vi "Email Worker (Tester).vi"(10 "Message Cluster":T1, 11 "Send Email?":bool) -> ()   [LabVIEW 2019]
doc: "Assembles the components of the message cluster into a more human-friendly email body message. Passes this, a constructed subject line, and the distribution list the Send Email subvi"
uses:
  Globals and Definitions/Initialization Globals.vi
  a5bfeb0e-6229-4f50-a4ef-3b1ccf936079.vi
  Globals and Definitions/System Message.ctl
panel:
  out "Receipients":string[](array[string])
  out "Message Subject Line":string
  out "Message Body":string
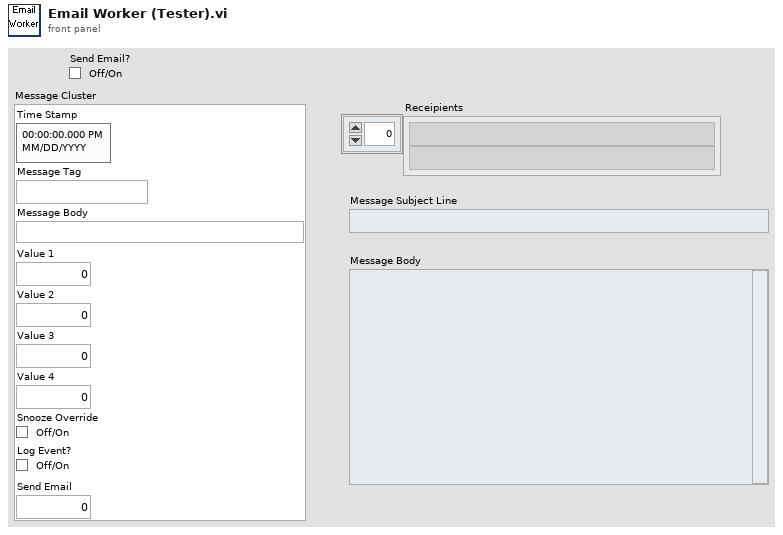
[diagram p1: front panel]
types:
  T1 = typedef "System Message.ctl" = cluster{"Time Stamp":timestamp, "Message Tag":string, "Message Body":string, "Value 1":i32, "Value 2":i32, "Value 3":dbl, "Value 4":dbl, "Snooze Override":bool, "Log Event?":bool, "Send Email":i32}
  T2 = typedef "All Tab Controls RDv1.0.ctl" = cluster{"Watch Circle":T3, "FTP and AWS":T4, "Email Settings":T5, "Summary File":T6, "File Settings":T7, "Watchdog":T9, "PowGrp0":T10, "Scaling Factors Grp0":dbl[], "PowGrp0 Sampling":cluster{"PowGrp0 sample rate [Hz]":dbl, "PowGrp0 samples per channel":i32}, "Stbd 3 Phase Voltage Scaling":dbl[], "Stbd 3 Phase Current Scaling":dbl[]}
  T3 = typedef "Watch Circle.ctl" = cluster{"Set Point Lat (dd)":dbl, "Set Point Lon (dd)":dbl, "Yellow Alert Radius (m)":dbl, "Red Alert Radius (m)":dbl, "AWOL Radius (m)":dbl, "Yellow Alert Snooze (min)":dbl, "Red Alert Snooze (min)":dbl, "AWOL Radius Snooze (min)":dbl}
  T4 = typedef "AWS and FTP.ctl" = cluster{"AWS Access Key":string, "AWS Secret Key":string, "AWS Bucket":string, "Enable AWS Upload (Summary)":bool, "Enable FTP Upload":bool, "FTP Host":string, "FTP User":string, "FTP Password":string, "Destination write path (pos)":string, "Local file path (pos)":string, "Summary  Upload Interval pos (min)":i32, "Delete Local File After Upload":bool, "Destination write path (pow)":string, "Local file path (pow)":string, "Summary Upload Interval pow (min)":i32, "Enable AWS Upload (TDMS)":bool}
  T5 = typedef "Email Settings.ctl" = cluster{"Enable Alerts":bool, "Distribution List (comma separated) 1":string, "Distribution List (comma separated) 2":string, "Sender Email":string, "SMTP":string, "Username":string, "Password":string}
  T6 = typedef "Summary File.ctl" = cluster{"Enable CSV":bool, "CSV Averaging Time (Sec)":i32, "CSV Loop Delay (ms)":i32}
  T7 = typedef "File Settings.ctl" = cluster{"Config File Path":string, "Data Folder Path":string, "Raw Mode":string, "Raw Interval (min)":i32, "Raw Sampling Time (min)":i32, "TDMS File Write Interval":T8, "Default Filename":path, "Enable TDMS Save (3ph only)":bool}
  T8 = typedef "Enum_FileNewInterval.ctl" = enum16{"10 Min", "Hourly", "Daily", "Weekly", "Monthly"}
  T9 = typedef "Watchdog.ctl" = cluster{"Watchdog Period (ms)":u32, "Reset System on WD timeout":bool, "Enable RT Watchdog":bool}
  T10 = typedef "TDMS Constants.ctl" = cluster{"Channel Names":string[], "Channel Units":string[], "TDMS File Suffix":string, "Channel Datatype":string[]}
  T11 = typedef "MODAQ _FPGA VI Reference.ctl" = refnum<k20>
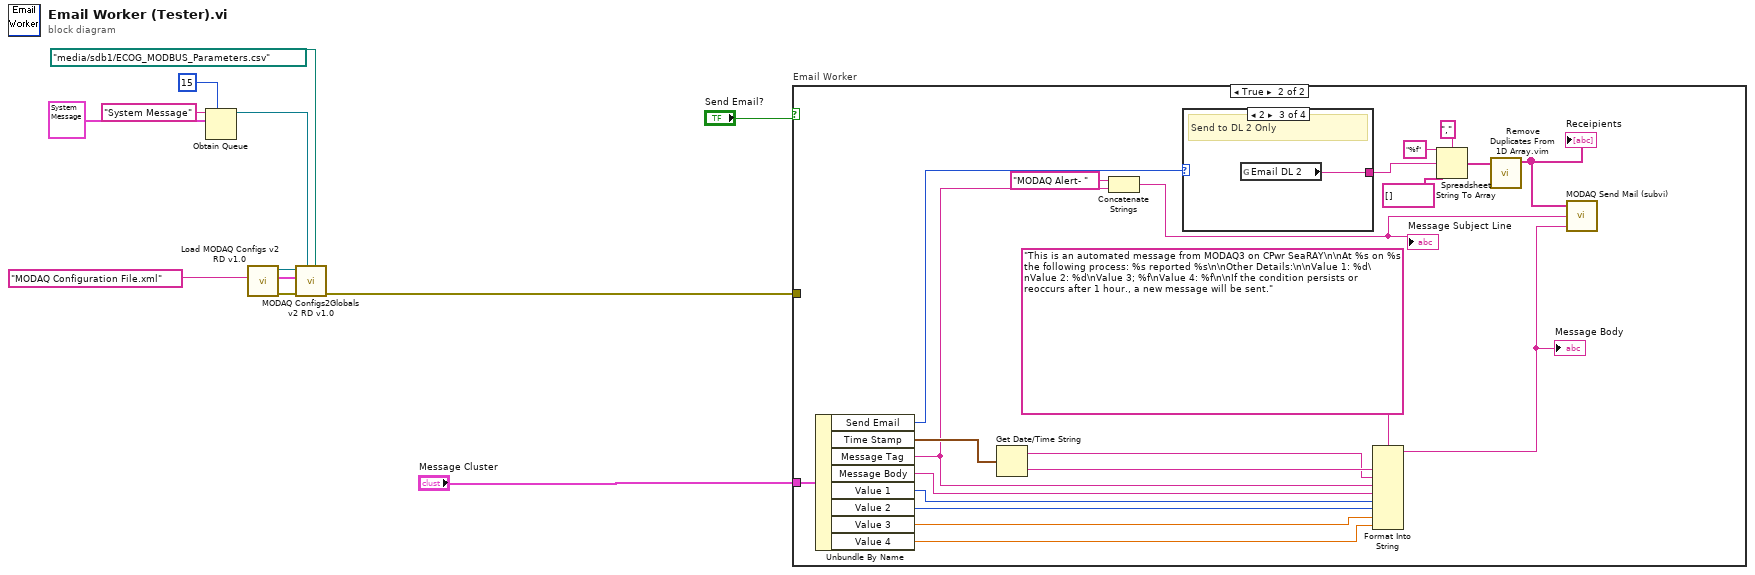
[diagram p0: block diagram]
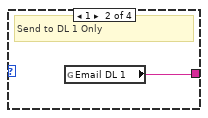
[diagram p4: hidden frame]
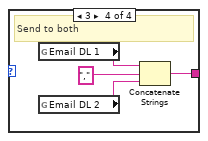
[diagram p5: hidden frame]
diagram:
  n1 = Obtain Queue(max queue size (-1, unlimited)=15, name (unnamed)="System Message", element data type=T1 {"Time Stamp"=timestamp(0 s since 1904-01-01), "Message Tag"="", "Message Body"="", "Value 1"=0, "Value 2"=0, "Value 3"=0.0, "Value 4"=0.0, "Snooze Override"=TRUE, "Log Event?"=TRUE, "Send Email"=0}) -> (queue out=w1:refnum<queue>)  [unwired: 2 in, 2 out]
  n2 = call "Load MODAQ Configs v2 RD v1.0.vi"("MODAQ Config Filename"="MODAQ Configuration File.xml") -> ("error out"=w8:errorcluster, "Configs out"=w6:T2, "FPGA Out"=w9:T11)  [unwired: 8 in]
  n3 = call "MODAQ Configs2Globals v2 RD v1.0.vi"("FPGA In"=w9, "Configs in"=w6, "error in"=w8, "Queue in"=w1, 5:path "/media/sdb1/ECOG_MODBUS_Parameters.csv" ("ECOG Modbus Parameters csv file")) -> ("error out"=w7:errorcluster)  [unwired: 4 in, 1 out]
  n4 = case "Email Worker" shown="True" "Send Email?" {
    tunnel: "Message Cluster" -> [_ w27]
    tunnel: w7 -> [_ _]
    frame False {
    }
    frame True {
      n5 = Unbundle By Name(w27) -> ("Send Email"=w26:i32, "Time Stamp"=w25:timestamp, "Message Tag"=w18:string, "Message Body"=w17:string, "Value 1"=w16:i32, "Value 2"=w15:i32, "Value 3"=w14:dbl, "Value 4"=w13:dbl)
      n6 = Get Date/Time String(seconds (now)=w25) -> (date string=w19:string, time string=w20:string)  [unwired: 2 in]
      n7 = Concatenate Strings("MODAQ Alert- " ("string"), w18) -> (w28:string)
      "Message Subject Line" <- w28
      n8 = case shown="2" w26 {
        tunnel: [_ w34 w35 w36] -> w30
        frame 0, Default {
        }
        frame 1 {
          # "Send to DL 1 Only"
          n9 = global read "Initialization Globals.vi" "Email DL 1"() -> (w34:string)
        }
        frame 2 {
          # "Send to DL 2 Only"
          n10 = global read "Initialization Globals.vi" "Email DL 2"() -> (w35:string)
        }
        frame 3 {
          # "Send to both"
          n11 = global read "Initialization Globals.vi" "Email DL 1"() -> (w39:string)
          n12 = global read "Initialization Globals.vi" "Email DL 2"() -> (w37:string)
          n13 = Concatenate Strings(w39, "," ("string"), w37) -> (w36:string)
        }
      }
      n14 = Format Into String(format string="This is an automated message from MODAQ3 on CPwr SeaRAY\n\nAt %s on %s the following process: %s reported %s\n\nOther Details:\n\nValue 1: %d\nValue 2: %d\nValue 3; %f\nValue 4: %f\n\nIf the condition persists or reoccurs after 1 hour., a new message will be sent." ("string"), w20, w19, w18, w17, w16, w15, w14, w13) -> (resulting string=w21:string)  [unwired: 2 in, 1 out]
      "Message Body" <- w21
      n15 = Spreadsheet String To Array(delimiter (Tab)=",", format string="%f", spreadsheet string=w30, array type (2D Dbl)=string[] []) -> (array=w24:string[])
      n16 = call "Remove Duplicates From 1D Array.vim"("array"=w24) -> ("array with duplicates removed"=w23:string[])  [unwired: 10 in]
      "Receipients" <- w23
      n17 = call "MODAQ Send Mail (subvi).vi"("Message"=w21, "Subject"=w28, "To"=w23) -> ()  [unwired: 1 out]
    }
  }
